vi "Destroy.vi"(8 "Error In":errorcluster, 11 "SFTP":refnum<class "SFTP.lvclass">) -> (0 "Error Out":errorcluster, 3 "lv-libssh2 Shared Library":path)   [LabVIEW 2017, in "Toolkit.lvlib" / "SFTP.lvclass"]
uses:
  SFTP.lvclass
  SFTP.lvclass/SFTP.ctl
  Toolkit.lvlib
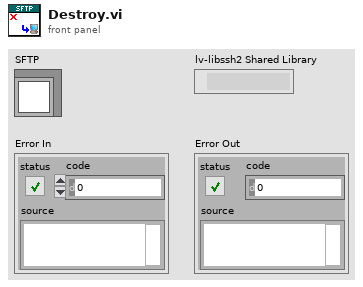
[diagram p1: front panel]
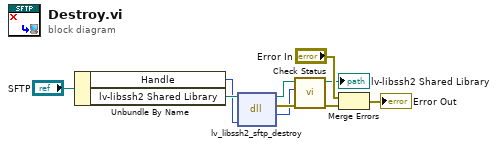
[diagram p0: block diagram]
diagram:
  n1 = Unbundle By Name("SFTP") -> ("Handle"=w7:u64, "lv-libssh2 Shared Library"=w8:path)
  n2 = dll-call lib="D:/Users/cfield/Code/Field R&D Services/SSH/LV-LIBSSH2/LabVIEW/trunk/src/Toolkit/Support/lv-libssh2.dll" fn="lv_libssh2_sftp_destroy"(path in=w8, "handle"=w7) -> (path out=w5:path, error out=w6:errorcluster, "status"=w2:i32)  [unwired: 3 in]
  n3 = call "Check Status.vi"("Error In"=w6, "Status"=w2, "lv-libssh2 Shared Library In"=w5) -> ("Error Out"=w3:errorcluster, "lv-libssh2 Shared Library Out"=→"lv-libssh2 Shared Library":path)  [unwired: 7 in]
  n4 = Merge Errors("Error In", w3) -> (→"Error Out":errorcluster)
